vi "PowerGuardSetFanMode.vi"(0 "error in (no error)":errorcluster, 2 "Fan Mode":u32(ring)=3 items=["FAN_MODE_OFF"=1, "FAN_MODE_ON"=2, "FAN_MODE_AUTO"=3], 3 "Device In":u64) -> (7 "error out":errorcluster, 10 "Device Out":u64)   [LabVIEW 2012, in "Phidget Power Guard.lvlib"]
doc: "${FanMode:Header}"
uses:
  <instrlib>/Phidgets/Phidget Power Guard/Phidget Power Guard.lvlib
  <instrlib>/Phidgets/Phidget Common/Phidget Common.lvlib
  phidget22.dll
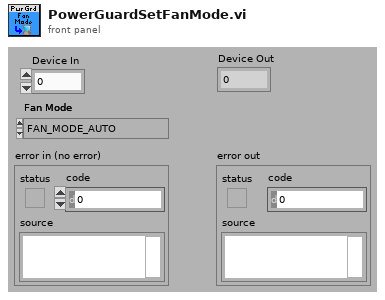
[diagram p1: front panel]
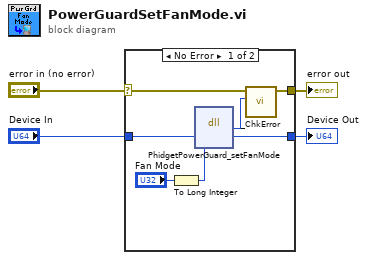
[diagram p0: block diagram]
diagram:
  n1 = case shown="No Error" "error in (no error)" {
    selector: "error in (no error)" -> [w9 w13]
    tunnel: [w8 w13] -> w3
    tunnel: "Device In" -> [w11 w12]
    tunnel: [w10 w12] -> w1
    frame No Error {
      n2 = To Long Integer(number="Fan Mode") -> (32bit integer=w5:i32)
      n3 = dll-call lib="phidget22.*" fn="PhidgetPowerGuard_setFanMode"("phid"=w11, "interval"=w5) -> ("return type"=w7:i32, "phid"=w10:u64)  [unwired: 4 in, 2 out]
      n4 = call <instrlib>:"_ChkError.vi"("Return Code"=w7, "error in (no error)"=w9) -> ("error out"=w8:errorcluster)  [unwired: 9 in]
    }
    frame Error {
    }
  }
  "error out" <- w3
  "Device Out" <- w1
